vi "GetNI_SaveToFile_25.vi"(0 "Digitizer Settings":T8={"Digitizer delay (us) "=0.0, "rf points per line"=2048, "lines per plane"=128, "Samp Rate (Hz)"=100000000.0, "Additional dig delay (us)"=0.0, "Voltage Scale"=0.4, "Pre-Looks"=0, "Offset delay (us)"=0.0, "bits A/D"=8, "Avg Num"=1, "DigTimeOut"=5.0, "Rel Dig Delay"=0.0, "Dig Ch"=0, "LeCroyCluster"={"LeCroy Channels"=[TRUE, FALSE, FALSE, FALSE], "LC read pt offset"=0.0, "Sweep Avg"=FALSE}, "Main Digitizer"=enum."NI Digitizer", "Dig Config"=enum."Single channel", "Digitizer ID Cluster"={"Acqiris/Alazar/SP ID"=[], "NI Instr Handles"=[], "LeCroy VISA"="", "GaGe Handle"={"Handle"=0, "Sample size"=0, "Resolution"=0, "Offset"=0, "Channels"=0, "Boards"=0}, "ATS Ref"="ATS9350", "Acqiris Address"=["PCI::INSTR0"], "ADQRef"=refnum, "adq_cu_ptr"=refnum}, "Trigger Settings"={"Trig Source"=1, "Trig Coupling"=0, "Trig Slope"=0, "Level (mV)"=1500.0}, "Bulk Acq"=FALSE, "Bulk Start Indexes"=[], "Data Ref RF"=refnum, "NI ID/Channel"=[], "Total Dig CH"=1, "Xtra Ann Trig delay (us)"=10.0, "Fix Z Delay?"=FALSE, "One Way Transmission?"=FALSE, "Data Ref Log"=refnum} {"Trigger Settings"."Trig Slope" items=["Positive", "Negative"]; "Trigger Settings"."Level (mV)" format="%.2f"; "Trigger Settings"."Trig Coupling" items=["DC 1 MOhm", "AC 1 MOhm", "DC 50 Ohm", "AC 50 Ohm"]; "Trigger Settings"."Trig Source" items=["Chan 1", "External"]; "Rel Dig Delay" format="%.2f"; "DigTimeOut" format="%.2f"; "Avg Num" min=1; "Offset delay (us)" format="%.2f"; "Additional dig delay (us)" format="%.2f"; "Digitizer delay (us)" format="%.2f"}, 2 "Ann Array Params":T1={"Synth Foc?"=FALSE, "Focal Zones"=41, "Switch T/R"=0, "Trans Geometry (mm)"={"Transducer"=0, "Geo Focus"=12.0, "a (radius)"=3.0, "# of rings"=5, "kerf space "=0.1, "Center Freq"=12.0}, "Sub Ap Excite?"=FALSE, "Full Array Scan?"=FALSE, "Xmt/Rcv"={"XMIT"=[TRUE, TRUE, TRUE, TRUE, TRUE], "RCV"=[TRUE, TRUE, TRUE, TRUE, TRUE]}, "PulseSpacing (us)"=0.0, "Xmit Ring"=0, "XMIT CHS"=0, "RCV CHS"=0, "GPU?"=FALSE, "Save TIFF?"=FALSE, "downfactor"=1, "RCV 1CH"=0} {"RCV 1CH" items=["All", "1", "2", "3", "4", "5"]; "Trans Geometry (mm)"."Transducer" items=["6D 12R 40 MHz"=0, "10D 31R 20 MHz"=1, "10D 23R 20 MHz"=2, "6D 23R 40 MHz"=3, "4.5D 10.7R 40 MHz"=4, "9D 23.5R 20 MHz"=5, "9D 25.8R 20MHz"=6, "Enter"=99]; "Switch T/R" min=1 max=5 step=1}, 6 "Motion Settings":T4={"No Motion?"=FALSE, "Motion System"=enum."NI 735x", "Motion Bd ID"=1, "Motion Profile"="SMAC1", "# Axis"=1, "Reverse Z axis?"=TRUE, "SMAC Axis"=0, "scan pair"=enum."y-(x) scan", "RT fps"=6.0, "Steps per mm"=[1000, 1000, 1000, 1000], "Motor Parameters"={"velocity ct/s"=[10000.0, 10000.0, 10000.0, 50000.0], "accel ct/s^2"=[50000.0, 50000.0, 50000.0, 200000.0]}, "One Way Scan"=FALSE, "Reverse One Way Scan"=FALSE, "Global Position (mm)"=[], "Plane"=0, "Distance between\nscan lines (um)"=0.0, "Distance between\nscan planes (um)"=0.0, "number of scan planes"=1, "Total steps in line"=0, "Xtra plane\ndistance  (um)"=100, "Xtra planes "=1, "Add Axis"=FALSE, "overshoot cts"=200, "BKPT Shift"=0, "Scan Start Time (ms)"=0, "ESP VISA"="GPIB::1::INSTR", "3rd Axis"=1, "GL Ref Out"=refnum, "Galil Address"=""} {"3rd Axis" items=["x", "y", "z", "w"]; "Xtra planes" min=1; "Xtra plane\ndistance  (um)" min=0; "Distance between\nscan planes (um)" format="%.2f"; "Distance between\nscan lines (um)" format="%.2f"; "SMAC Axis" items=["None"=0, "Axis 1"=1, "Axis 2"=2, "Axis 3"=3, "Axis 4"=4, "Axis 5"=5, "Axis 6"=6, "Axis 7"=7, "Axis 8"=8, "Vector Space 1"=17, "Vector Space 2"=18, "Vector Space 3"=19, "Vector Space 4"=20]; "Motion Bd ID" min=1 max=32 step=1}, 7 "errorin":errorcluster, 8 "File Array":string[](array[string]), 10 "lines per plane":i32, 15 "Reverse?":bool) -> (17 "Raw VGain (scale)":dbl, 18 "Gain Array":T12(array[cluster]), 21 "VGain (dB)":dbl, 27 "error out":errorcluster)   [LabVIEW 2022 SP3]
uses:
  -DigitizerRoutines/DigitizerSettings.ctl
  -DigitizerRoutines/Digitizer.ctl
  -DigitizerRoutines/DigConfig.ctl
  -DigitizerRoutines/DigitizerID.ctl
  C:/Windows/System32/ADQAPI_dotNet_helper.dll
  Motion Controllers/NI_controller/-NI_MotionRoutines/MotionParameters.ctl
  Motion Controllers/NI_controller/-NI_MotionRoutines/MotionSys.ctl
  Motion Controllers/-MotionRoutines/ScanAxis.ctl
  Motion Controllers/-MotionRoutines/3rdAxis.ctl
  Annular Array/-AnnularRoutines/AnnularArray.ctl
  Annular Array/-AnnularRoutines/TransGeometry.ctl
  Annular Array/-AnnularRoutines/ArrayGeometry.ctl
  <instrlib>/niScope/Acquire/Fetch/niScope Multi Fetch Binary 8.vi
  Motion Controllers/-MotionRoutines/MotionGlobals.vi
  -ScanSystem/DataHandling/ReverseDataI8.vi
panel:
  out "read time":u32
  out "save time":u32
  out "Numeric":i32
  # "1-D and 2-D B scan settings"
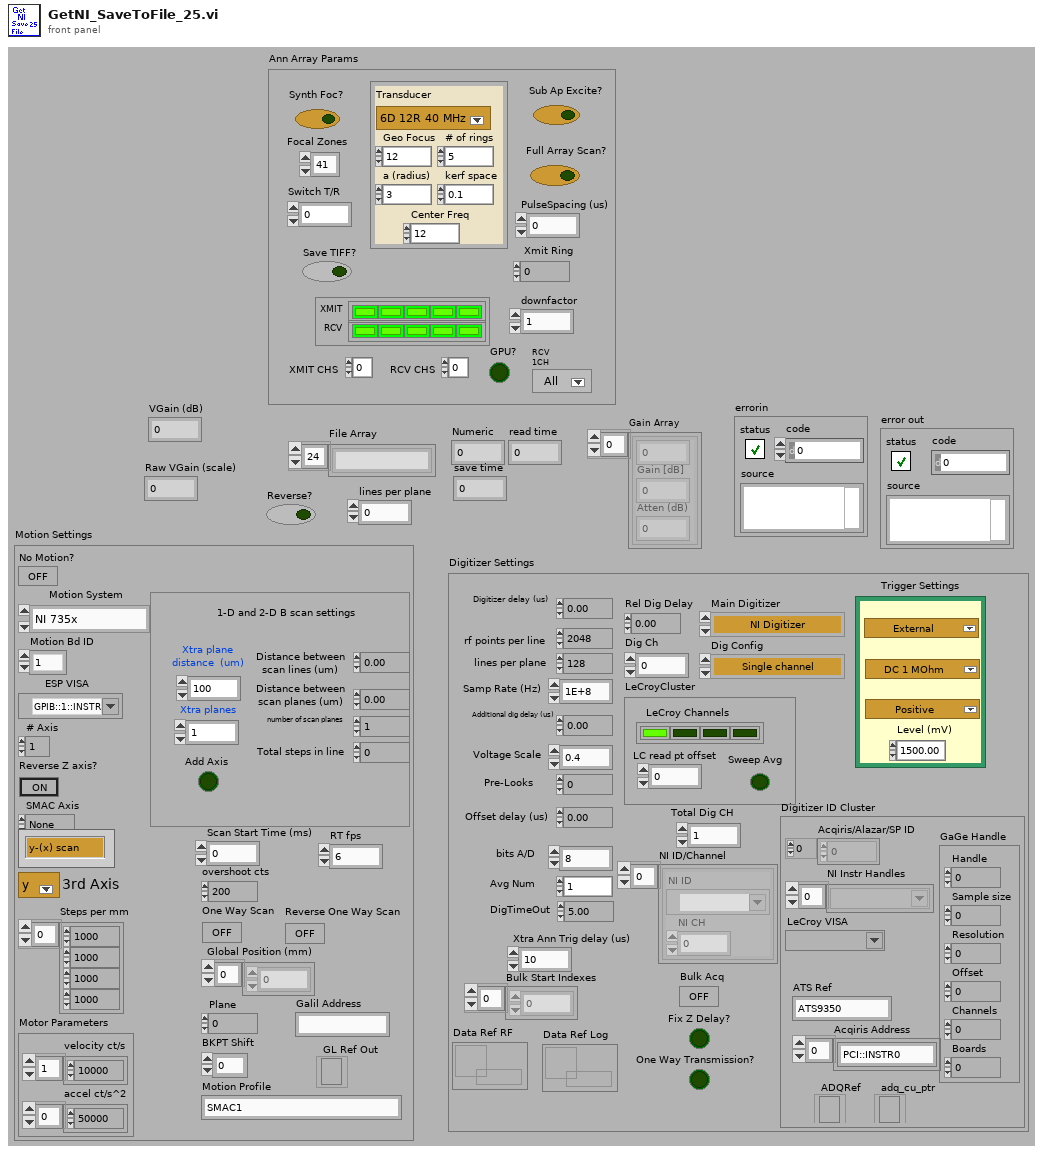
[diagram p1: front panel]
types:
  T1 = typedef "AnnularArray.ctl" = cluster{"Synth Foc?":bool, "Focal Zones":i16, "Switch T/R":i16, "Trans Geometry (mm)":T2, "Sub Ap Excite?":bool, "Full Array Scan?":bool, "Xmt/Rcv":cluster{"XMIT":bool[], "RCV":bool[]}, "PulseSpacing (us)":sgl, "Xmit Ring":i32, "XMIT CHS":u8, "RCV CHS":u8, "GPU?":bool, "Save TIFF?":bool, "downfactor":i32, "RCV 1CH":u16}
  T2 = typedef "TransGeometry.ctl" = cluster{"Transducer":T3, "Geo Focus":dbl, "a (radius)":dbl, "# of rings":i32, "kerf space ":dbl, "Center Freq":dbl}
  T3 = typedef "ArrayGeometry.ctl" = u16
  T4 = typedef "MotionParameters.ctl" = cluster{"No Motion?":bool, "Motion System":T5, "Motion Bd ID":u8, "Motion Profile":string, "# Axis":i8, "Reverse Z axis?":bool, "SMAC Axis":u16, "scan pair":T6, "RT fps":sgl, "Steps per mm":i32[], "Motor Parameters":cluster{"velocity ct/s":dbl[], "accel ct/s^2":dbl[]}, "One Way Scan":bool, "Reverse One Way Scan":bool, "Global Position (mm)":dbl[], "Plane":i32, "Distance between\nscan lines (um)":sgl, "Distance between\nscan planes (um)":sgl, "number of scan planes":i32, "Total steps in line":i32, "Xtra plane\ndistance  (um)":i32, "Xtra planes ":i32, "Add Axis":bool, "overshoot cts":i32, "BKPT Shift":i32, "Scan Start Time (ms)":u32, "ESP VISA":refnum<visa-resource-name>, "3rd Axis":T7, "GL Ref Out":refnum<k7>, "Galil Address":string}
  T5 = typedef "MotionSys.ctl" = enum16{"MM3000", "NI 735x", "Newport ESP", "No Motion Card", "Galil"}
  T6 = typedef "ScanAxis.ctl" = enum16{"y-(x) scan", "x-(y) scan", "z-(x) scan", "z-(y) scan", "y-(z) scan", "x-(z) scan", "w-(x) scan", "w-(y) scan", "w-(z) scan", "x-(w) scan", "y-(w) scan", "z-(w) scan"}
  T7 = typedef "3rdAxis.ctl" = u16
  T8 = typedef "DigitizerSettings.ctl" = cluster{"Digitizer delay (us) ":dbl, "rf points per line":i32, "lines per plane":i32, "Samp Rate (Hz)":dbl, "Additional dig delay (us)":dbl, "Voltage Scale":dbl, "Pre-Looks":i32, "Offset delay (us)":dbl, "bits A/D":i8, "Avg Num":i32, "DigTimeOut":sgl, "Rel Dig Delay":sgl, "Dig Ch":i32, "LeCroyCluster":cluster{"LeCroy Channels":bool[], "LC read pt offset":dbl, "Sweep Avg":bool}, "Main Digitizer":T9, "Dig Config":T10, "Digitizer ID Cluster":T11, "Trigger Settings":cluster{"Trig Source":u16, "Trig Coupling":u16, "Trig Slope":u16, "Level (mV)":dbl}, "Bulk Acq":bool, "Bulk Start Indexes":i32[], "Data Ref RF":refnum<data-value>, "NI ID/Channel":cluster{"NI ID":refnum<k15>, "NI CH":i32}[], "Total Dig CH":i32, "Xtra Ann Trig delay (us)":dbl, "Fix Z Delay?":bool, "One Way Transmission?":bool, "Data Ref Log":refnum<data-value>}
  T9 = typedef "Digitizer.ctl" = enum16{"Acqiris Digitizer", "NI Digitizer", "LeCroy", "GaGe", "AlazarTech", "No Digitizer", "Teledyne"}
  T10 = typedef "DigConfig.ctl" = enum16{"Single channel", "2 Chans w/ 2 Acqiris", "2 Chans w/ 1 Acqiris", "5-CH Pulser New", "5-CH pulser w/ ann array", "5-pass style ann array", "Empty"}
  T11 = typedef "DigitizerID.ctl" = cluster{"Acqiris/Alazar/SP ID":u32[], "NI Instr Handles":refnum<k15>[], "LeCroy VISA":refnum<visa-resource-name>, "GaGe Handle":cluster{"Handle":u32, "Sample size":u32, "Resolution":i32, "Offset":i32, "Channels":u32, "Boards":u32}, "ATS Ref":string, "Acqiris Address":string[], "ADQRef":refnum<k24>, "adq_cu_ptr":refnum<k24>}
  T12 = cluster{sgl, "Gain [dB]  ":sgl, "Atten (dB)":sgl}[]
  T13 = cluster{"gain":dbl, "wfm":i8[][], "max queue size (-1, unlimited)":i32}
  T14 = cluster{"actualSamples":i32, "absoluteInitialX":dbl, "relativeInitialX":dbl, "xIncrement":dbl, "offset":dbl, "gain":dbl, "reserved1":dbl, "reserved2":dbl}[]
  T15 = cluster{"actualSamples":i32, "absoluteInitialX":dbl, "relativeInitialX":dbl, "xIncrement":dbl, "offset":dbl, "gain":dbl, "reserved1":dbl, "reserved2":dbl}
  T16 = enum16{"open", "replace", "create", "open or create", "replace or create", "replace or create with confirmation"}
  T17 = cluster{sgl, "Gain [dB]  ":sgl, "Atten (dB)":sgl}
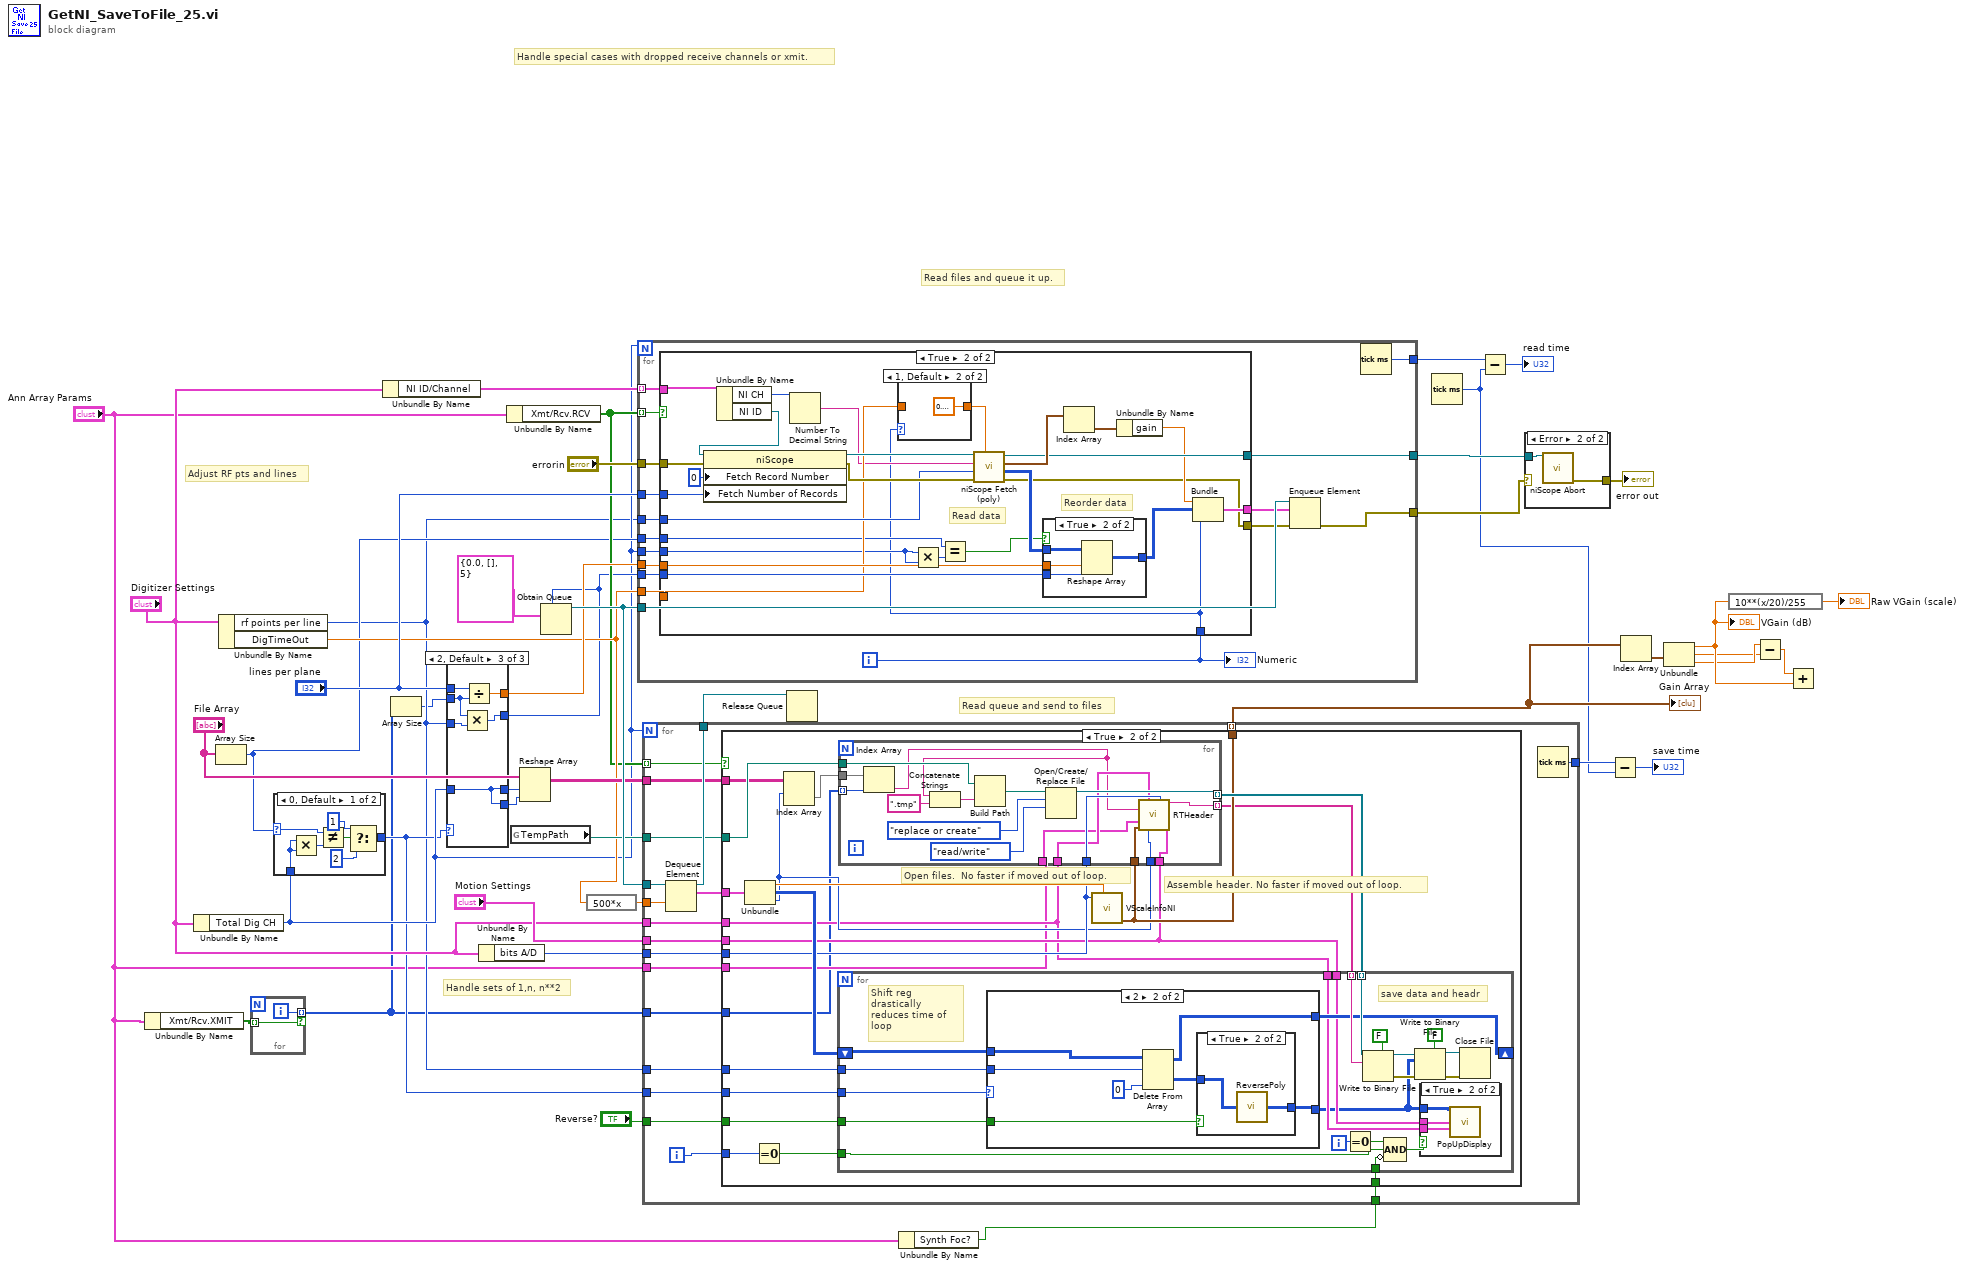
[diagram p0: block diagram]
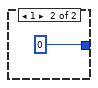
[diagram p2: hidden frame]
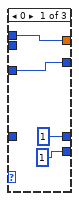
[diagram p3: hidden frame]
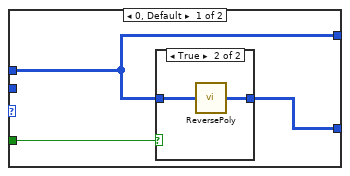
[diagram p7: hidden frame]
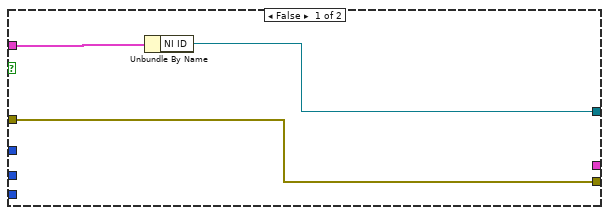
[diagram p11: hidden frame]
diagram:
  # "Adjust RF pts and lines"
  # "Handle special cases with dropped receive channels or xmit."
  # "Handle sets of 1,n, n**2"
  # "Read files and queue it up."
  # "Read queue and send to files"
  n1 = Unbundle By Name("Ann Array Params") -> ("Xmt/Rcv.XMIT"=w3:bool[])
  n2 = Unbundle By Name("Digitizer Settings") -> ("Total Dig CH"=w8:i32)
  n3 = Array Size(array="File Array") -> (size(s)=w9:i32)
  n4 = Unbundle By Name("Digitizer Settings") -> ("rf points per line"=w6:i32, "DigTimeOut"=w15:sgl)
  n5 = for {
    tunnel: w3 -> [w46] mode=indexing
    tunnel: [w45] -> w2 mode=indexing if=w46
    i -> [w45]
  }
  n6 = case shown="0, Default" w9 {
    selector: w9 -> [w53 _]
    tunnel: w8 -> [w52 _]
    tunnel: [w51 0] -> w7
    frame 0, Default {
      n7 = Multiply(x=w52, y=w52) -> (x*y=w49:i32)
      n8 = Not Equal?(x=w53, y=w49) -> (x != y?=w50:bool)
      n9 = Select(t=1, s=w50, f=2) -> (s? t:f=w51:i32)
    }
    frame 1 {
    }
  }
  n10 = Unbundle By Name("Digitizer Settings") -> ("NI ID/Channel"=w12:cluster{"NI ID":refnum<k15>, "NI CH":i32}[])
  n11 = Array Size(array=w2) -> (size(s)=w1:i32)
  n12 = case shown="2, Default" w7 {
    tunnel: [1 w60 w64] -> w23
    tunnel: [w55 w59 w65] -> w10
    tunnel: [w57 w61 w66] -> w20
    tunnel: "lines per plane" -> [w57 w61 w67]
    tunnel: [1 w60 w64] -> w21
    tunnel: w8 -> [_ w60 w64]
    tunnel: w6 -> [w55 w59 w63]
    tunnel: w1 -> [_ _ w62]
    frame 0 {
    }
    frame 1 {
    }
    frame 2, Default {
      n13 = Multiply(x=w62, y=w63) -> (x*y=w65:i32)
      n14 = Divide(x=w67, y=w62) -> (x/y=w66:dbl)
    }
  }
  n15 = Unbundle By Name("Digitizer Settings") -> ("bits A/D"=w16:i8)
  n16 = Unbundle By Name("Ann Array Params") -> ("Xmt/Rcv.RCV"=w13:bool[])
  n17 = global read "MotionGlobals.vi" "TempPath"() -> (w17:path)
  n18 = Reshape Array("File Array", w23, w21) -> (w18:string[][])
  n19 = Obtain Queue(max queue size (-1, unlimited)=w10, element data type=T13 {"gain"=0.0, "wfm"=[], "max queue size (-1, unlimited)"=5}) -> (queue out=w33:refnum<queue>)  [unwired: 3 in, 2 out]
  n20 = expression code="500*x"(w15) -> (w19:sgl)
  n21 = for {
    N: w8 -> [_]
    tunnel: w15 -> [w71]
    tunnel: w6 -> [w81]
    tunnel: "errorin" -> [w84]
    tunnel: "lines per plane" -> [w83]
    tunnel: [w82] -> w42
    tunnel: w33 -> [w80]
    tunnel: [w73] -> w32
    tunnel: [w78] -> w31
    tunnel: w20 -> [w77]
    tunnel: w10 -> [w76]
    tunnel: w9 -> [w75]
    tunnel: w13 -> [w70] mode=indexing
    tunnel: w12 -> [w69] mode=indexing
    tunnel: w8 -> [w68]
    i -> [w72]
    n22 = case shown="True" w70 {
      tunnel: w84 -> [w87 w114]
      tunnel: w83 -> [_ w109]
      tunnel: [w85 w108] -> w82
      tunnel: w81 -> [_ w106]
      tunnel: [_ w104] -> w79
      tunnel: w77 -> [_ w102]
      tunnel: w76 -> [_ w101]
      tunnel: w75 -> [_ w90]
      tunnel: [w87 w99] -> w74
      tunnel: w72 -> [_ w88]
      tunnel: w71 -> [_ w98]
      tunnel: w69 -> [w86 w96]
      tunnel: w68 -> [_ w91]
      frame False {
        n23 = Unbundle By Name(w86) -> ("NI ID"=w85:refnum<k15>)
      }
      frame True {
        # "Reorder data"
        # "Read data"
        n24 = Unbundle By Name(w96) -> ("NI CH"=w95:i32, "NI ID"=w93:refnum<k15>)
        n25 = property class="niScope"(reference=w93, error in=w114, "Fetch Record Number"=0, "Fetch Number of Records"=w109) -> (reference out=w107:refnum<k15>, error out=w113:errorcluster)
        n26 = Number To Decimal String(number=w95) -> (decimal integer string=w94:string)  [unwired: 1 in]
        n27 = case shown="1, Default" w88 {
          tunnel: w98 -> [w115 _]
          tunnel: [w115 sgl 0.1 ("DigTimeOut")] -> w97
          frame 0 {
          }
          frame 1, Default {
          }
        }
        n28 = Multiply(x=w91, y=w91) -> (x*y=w92:i32)
        n29 = Equal?(x=w90, y=w92) -> (x = y?=w89:bool)
        n30 = call-poly <instrlib>:"niScope Fetch (poly).vi"("timeout"=w97, "error in"=w113, "numSamples"=w106, "channels"=w94, "instrument handle"=w107) -> ("error out"=w99:errorcluster, "wfm"=w103:i8[][], "wfm info"=w112:T14, "instrument handle out"=w108:refnum<k15>)  [unwired: 3 out]
        n31 = case shown="True" w89 {
          tunnel: w101 -> [_ w121]
          tunnel: w103 -> [w117 w120]
          tunnel: [w117 w119] -> w100
          tunnel: w102 -> [_ w118]
          frame False {
          }
          frame True {
            n32 = Reshape Array(w120, w118, w121) -> (w119:i8[][])
          }
        }
        n33 = Index Array(array=w112) -> (element=w111:T15)  [unwired: 1 in]
        n34 = Unbundle By Name(w111) -> ("gain"=w105:dbl)
        n35 = Bundle("gain"=w105, "wfm"=w100, w88) -> (w104:cluster{"gain":dbl, "wfm":i8[][], i32})  [unwired: 1 in]
      }
    }
    n36 = Enqueue Element(queue=w80, element=w79, error in (no error)=w74) -> (error out=w73:errorcluster)  [unwired: 1 in, 2 out]
    n37 = Tick Count (ms)() -> (millisecond timer value=w78:u32)
    "Numeric" <- w72
  }
  n38 = Unbundle By Name("Ann Array Params") -> ("Synth Foc?"=w5:bool)
  n39 = for {
    N: w8 -> [_]
    tunnel: w6 -> [w140]
    tunnel: "Reverse?" -> [w135]
    tunnel: [w131] -> w34 mode=indexing
    tunnel: w33 -> [w139]
    tunnel: [w137] -> w25
    tunnel: [w136] -> w30
    tunnel: w7 -> [w134]
    tunnel: w19 -> [w133]
    tunnel: w18 -> [w130]
    tunnel: w17 -> [w132]
    tunnel: w16 -> [w129]
    tunnel: "Digitizer Settings" -> [w128]
    tunnel: "Motion Settings" -> [w127]
    tunnel: w13 -> [w126] mode=indexing
    tunnel: w5 -> [w124]
    tunnel: "Ann Array Params" -> [w123]
    tunnel: w2 -> [w122]
    i -> [w125]
    n40 = Dequeue Element(queue=w139, timeout in ms (-1)=w133) -> (queue out=w137:refnum<queue>, element=w138:T13)  [unwired: 1 in, 2 out]
    n41 = case shown="True" w126 {
      tunnel: w140 -> [_ w161]
      tunnel: w138 -> [_ w160]
      tunnel: w135 -> [_ w158]
      tunnel: w134 -> [_ w157]
      tunnel: w132 -> [_ w154]
      tunnel: [_ w153] -> w131
      tunnel: w130 -> [_ w151]
      tunnel: w129 -> [_ w150]
      tunnel: w128 -> [_ w146]
      tunnel: w127 -> [_ w147]
      tunnel: w125 -> [_ w148]
      tunnel: w124 -> [_ w144]
      tunnel: w123 -> [_ w143]
      tunnel: w122 -> [_ w141]
      frame False {
      }
      frame True {
        # "Open files.  No faster if moved out of loop."
        # "Assemble header. No faster if moved out of loop."
        n42 = Unbundle(w160) -> ("gain"=w159:dbl, "wfm"=w156:i8[][], "max queue size (-1, unlimited)"=w149:i32)
        n43 = Equal To 0?(x=w148) -> (x = 0?=w145:bool)
        n44 = Index Array(array=w151, index (row)=w149) -> (element=w142:string[])  [unwired: 1 in]
        n45 = call "VScaleInfoNI.vi"("A/D bits"=w150, "gain"=w159) -> ("Voltage Scale"=w153:T17)  [unwired: 5 in, 3 out]
        n46 = for {
          tunnel: [w173] -> w155 mode=indexing
          tunnel: w154 -> [w172]
          tunnel: w153 -> [w171]
          tunnel: [w170] -> w152 mode=indexing
          tunnel: w150 -> [w169]
          tunnel: w146 -> [w168]
          tunnel: w147 -> [w167]
          tunnel: w149 -> [w166]
          tunnel: w143 -> [w165]
          tunnel: w142 -> [w164]
          tunnel: w141 -> [w162] mode=indexing
          n47 = Index Array(array=w164, index=w162) -> (element=w163:string)
          n48 = Concatenate Strings(w163, ".tmp") -> (w174:string)
          n49 = Build Path(base path=w172, name or relative path=w174) -> (appended path=w178:path)
          n50 = Open/Create/Replace File(file path (use dialog)=w178, operation (0:open)=T16."replace or create", access (0:read/write)=enum16{"read/write", "read-only", "write-only"}."read/write") -> (refnum out=w173:refnum<file>)  [unwired: 1 in, 4 out]
          n51 = call "RTHeader.vi"("Digitizer Settings"=w168, "Dig Word Size"=w169, "File Name In"=w163, "Ann Array Params"=w165, "Votage scaling"=w171, "Pulser Channel"=w166, "Motion Settings"=w167) -> ("Header String Out"=w170:string)  [unwired: 7 in, 1 out]
        }
        n52 = for {
          tunnel: w152 -> [w197] mode=indexing
          tunnel: w158 -> [w196]
          tunnel: w155 -> [w190] mode=indexing
          tunnel: w161 -> [w195]
          tunnel: w157 -> [w193]
          shift-right: [w187] -> _
          shift-left: w156 -> [w194]
          tunnel: w145 -> [w182]
          tunnel: w147 -> [w186]
          tunnel: w146 -> [w185]
          tunnel: w144 -> [w179]
          i -> [w183]
          # "Shift reg drastically reduces time of loop"
          # "save data and headr"
          n53 = case shown="2" w193 {
            tunnel: w196 -> [w205 w213]
            tunnel: [w204 w214] -> w184
            tunnel: w195 -> [_ w210]
            tunnel: w194 -> [w203 w212]
            tunnel: [w203 w211] -> w187
            frame 0, Default {
              n54 = case shown="True" w205 {
                tunnel: [w206 w208] -> w204
                tunnel: w203 -> [w206 w207]
                frame False {
                }
                frame True {
                  n55 = call-poly "ReversePoly.vi"("Array in"=w207) -> ("Array out"=w208:i8[][])
                }
              }
            }
            frame 2 {
              n56 = Delete From Array(array=w212, length=w210, index (col)=0 ("index (row)")) -> (deleted portion=w215:i8[][], array with subset deleted=w211:i8[][])  [unwired: 1 in]
              n57 = case shown="True" w213 {
                tunnel: [w216 w218] -> w214
                tunnel: w215 -> [w216 w217]
                frame False {
                }
                frame True {
                  n58 = call-poly "ReversePoly.vi"("Array in"=w217) -> ("Array out"=w218:i8[][])
                }
              }
            }
          }
          n59 = Equal To 0?(x=w183) -> (x = 0?=w180:bool)
          n60 = Write to Binary File(file (use dialog)=w190, data=w197, 5:FALSE ("prepend array or string size? (T)")) -> (refnum out=w189:refnum<file>, error out=w188:errorcluster)  [unwired: 3 in, 1 out]
          n61 = Compound Arithmetic op=AND(w180, w182, invert w179) -> (w181:bool)
          n62 = Write to Binary File(file (use dialog)=w189, data=w184, error in=w188, 5:FALSE ("prepend array or string size? (T)")) -> (refnum out=w192:refnum<file>, error out=w191:errorcluster)  [unwired: 2 in, 1 out]
          n63 = case shown="True" w181 {
            tunnel: w186 -> [_ w202]
            tunnel: w185 -> [_ w201]
            tunnel: w184 -> [_ w200]
            frame False {
            }
            frame True {
              n64 = call "PopUpDisplay.vi"("Data"=w200, "Motion Settings In"=w202, "Digitizer Settings"=w201) -> ()  [unwired: 13 in]
            }
          }
          n65 = Close File(refnum=w192, error in=w191) -> ()  [unwired: 2 out]
        }
      }
    }
    n66 = Tick Count (ms)() -> (millisecond timer value=w136:u32)
  }
  "Gain Array" <- w34
  n67 = Release Queue(queue=w25) -> ()  [unwired: 2 in, 3 out]
  n68 = Tick Count (ms)() -> (millisecond timer value=w29:u32)
  n69 = Subtract(x=w31, y=w29) -> (x-y=→"read time":u32)
  n70 = case shown="Error" w32 {
    selector: w32 -> [w219 _]
    tunnel: w42 -> [_ w221]
    tunnel: [w219 w220] -> w43
    frame No Error {
    }
    frame Error {
      n71 = call <instrlib>:"niScope Abort.vi"("instrument handle"=w221) -> ("error out"=w220:errorcluster)  [unwired: 1 in, 13 out]
    }
  }
  "error out" <- w43
  n72 = Subtract(x=w30, y=w29) -> (x-y=→"save time":u32)
  n73 = Index Array(array=w34) -> (element=w41:T17)  [unwired: 1 in]
  n74 = Unbundle(w41) -> (w40:sgl, "Gain [dB]"=w38:sgl, "Atten (dB)"=w39:sgl)
  "VGain (dB)" <- w40
  n75 = expression code="10**(x/20)/255"(w40) -> (→"Raw VGain (scale)":sgl)
  n76 = Subtract(x=w39, y=w38) -> (x-y=w37:sgl)
  n77 = Add(x=w37, y=w40) -> ()  [unwired: 1 out]
